vi "Retrieve.vi"(8 "error in (no error)":errorcluster, 11 "Local in":refnum<class "Local.lvclass">) -> (0 "error out":errorcluster, 1 "Quem joga":string, 2 "Tabuleiro":T1, 3 "Local out":refnum<class "Local.lvclass">)   [LabVIEW 2019, in "Local.lvclass"]
uses:
  Local.lvclass
  controls/Tabuleiro.ctl
  MatchData/MatchData.lvclass
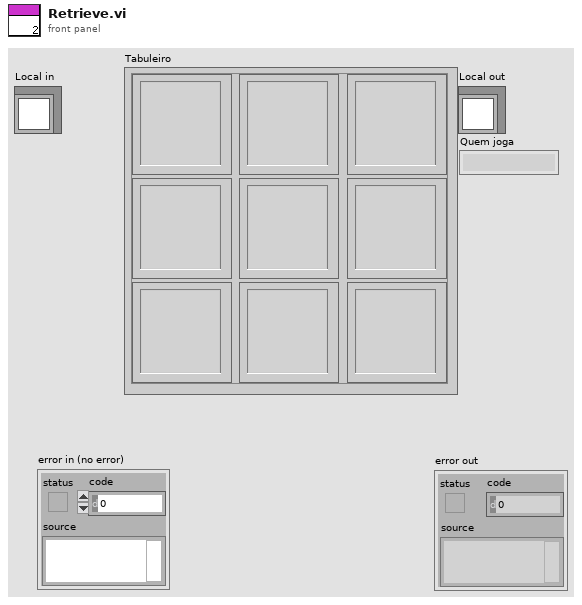
[diagram p1: front panel]
types:
  T1 = typedef "Tabuleiro.ctl" = cluster{"(0,0)":string, "(1,0)":string, "(0,1)":string, "(1,1)":string, "(2,0)":string, "(1,2)":string, "(2,2)":string, "(0,2)":string, "(2,1) ":string}
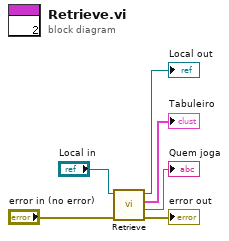
[diagram p0: block diagram]
diagram:
  n1 = call-parent "Retrieve.vi"("error in (no error)"="error in (no error)", "MatchData in"="Local in") -> ("error out"=→"error out":errorcluster, "Quem joga"=→"Quem joga":string, "Tabuleiro"=→"Tabuleiro":T1, "MatchData out"=→"Local out":refnum<class "Local.lvclass">)  [unwired: 6 in]
